vi "String-Boolean.vi"(9 "String in":string, 10 "Boolean in":bool) -> (1 "Boolean out":bool, 2 "String out":string)   [LabVIEW 2015]
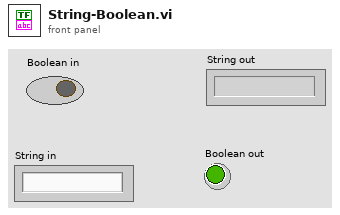
[diagram p1: front panel]
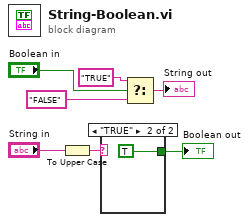
[diagram p0: block diagram]
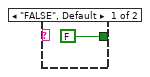
[diagram p2: hidden frame]
diagram:
  n1 = To Upper Case(1:"String in") -> (0:w2:string)
  n2 = case shown="\"TRUE\"" w2 {
    tunnel: [FALSE TRUE] -> w1
    frame "FALSE", Default {
    }
    frame "TRUE" {
    }
  }
  "Boolean out" <- w1
  n3 = Select(t="TRUE" ("String in 2"), s="Boolean in", f="FALSE" ("String in 2")) -> (s? t:f=→"String out":string)
